vi "AutonCSV.vi"(0 "Auton Array":dbl[][](array[numeric]), 5 "MeasuredHeading":dbl, 7 "LeftEncoder":dbl, 9 "RightEncoder":dbl, 11 "Kinect Array":dbl[](array[numeric])) -> (2 "Z Wrist Right out":dbl, 3 "Z Wrist Left out":dbl, 4 "Left Drive":dbl, 6 "Right Drive":dbl)   [LabVIEW 2011]
uses:
  <vilib>/addons/Kinect/Skeleton Vertex Index.ctl
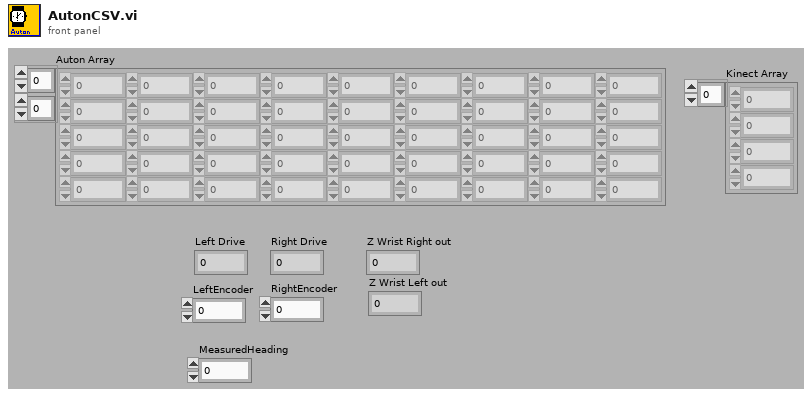
[diagram p1: front panel]
types:
  T1 = typedef "Skeleton Vertex Index.ctl" = i32
  T2 = cluster{"RightAxis":dbl, "LeftAxis":dbl, "RightHead":bool, "Left Head":bool, "Left Leg Out":bool, "Left Leg Forward":bool, "Left Leg Back":bool, "Right Leg Out":bool, "Right Leg Forward":bool, "Right Leg Back":bool}
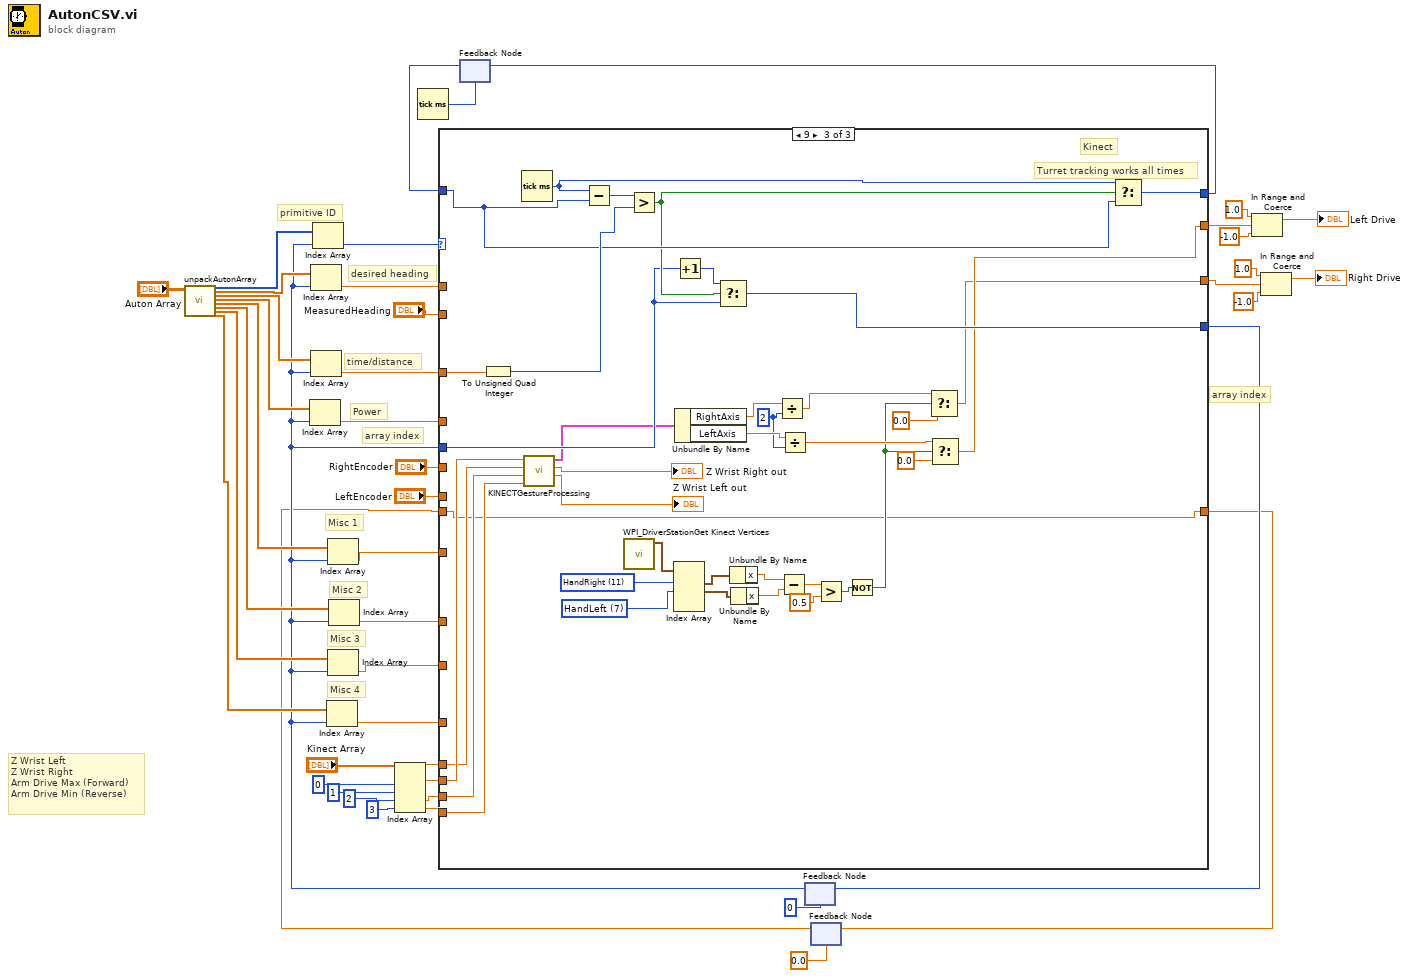
[diagram p0: block diagram]
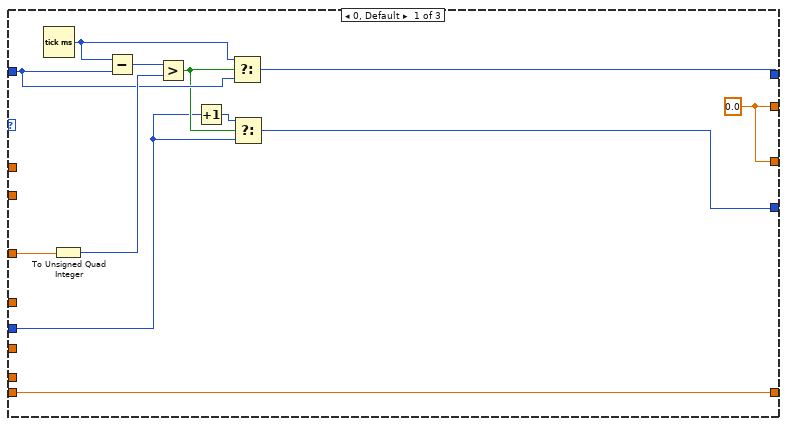
[diagram p2: hidden frame]
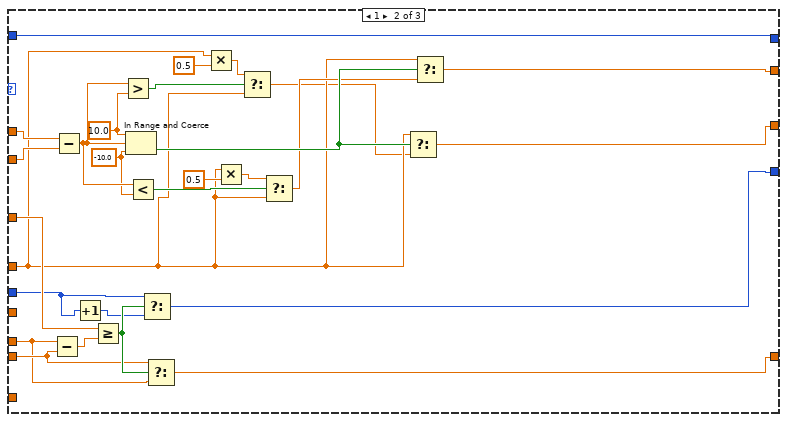
[diagram p3: hidden frame]
diagram:
  # "Misc 4"
  # "Misc 3"
  # "Misc 2"
  # "Misc 1"
  # "Z Wrist Left\nZ Wrist Right\nArm Drive Max (Forward)\nArm Drive Min (Reverse)"
  # "array index"
  # "array index"
  # "Power"
  # "desired heading"
  # "primitive ID"
  # "time/distance"
  n1 = call "unpackAutonArray.vi"("all rows"="Auton Array") -> ("Primitive"=w45:i16[], "Desired Heading"=w24:dbl[], "Time/Distance"=w23:dbl[], "Power"=w22:dbl[], "Misc 1"=w21:dbl[], "Misc 2"=w20:dbl[], "Misc 3"=w19:dbl[], "Misc 4"=w18:dbl[])  [unwired: 1 in, 18 out]
  n2 = Index Array(array="Kinect Array", index #1=0 ("index"), index #2=1 ("index"), index #3=2 ("index"), index #4=3 ("index")) -> (element #1=w7:dbl, element #2=w6:dbl, element #3=w5:dbl, element #4=w4:dbl)
  n3 = Tick Count (ms)() -> (millisecond timer value=w40:u32)
  n4 = feedback #1(w40) -> (w44:u32)
  n5 = feedback #2(0) -> (w16:i32)
  n6 = Index Array(array=w22, index=w16) -> (element=w42:dbl)
  n7 = Index Array(array=w24, index=w16) -> (element=w29:dbl)
  n8 = Index Array(array=w23, index=w16) -> (element=w43:dbl)
  n9 = Index Array(array=w45, index=w16) -> (element=w26:i16)
  n10 = Index Array(array=w18, index=w16) -> (element=w17:dbl)
  n11 = Index Array(array=w21, index=w16) -> (element=w25:dbl)
  n12 = Index Array(array=w19, index=w16) -> (element=w14:dbl)
  n13 = Index Array(array=w20, index=w16) -> (element=w15:dbl)
  n14 = feedback #3(0.0) -> (w2:dbl)
  n15 = case shown="9" w26 {
    tunnel: [w50 w81 w115] -> w27
    tunnel: w16 -> [w51 w61 w116]
    tunnel: [w58 w63 w123] -> w30
    tunnel: w44 -> [w55 w63 w120]
    tunnel: w43 -> [w48 w83 w114]
    tunnel: w29 -> [_ w80 _]
    tunnel: [w49 w77 w103] -> w38
    tunnel: [w49 w76 w102] -> w31
    tunnel: w42 -> [_ w65 _]
    tunnel: "LeftEncoder" -> [_ w59 _]
    tunnel: "MeasuredHeading" -> [_ w79 _]
    tunnel: w25 -> [_ _ _]
    tunnel: w17 -> [_ _ _]
    tunnel: w15 -> [_ _ _]
    tunnel: w14 -> [_ _ _]
    tunnel: "RightEncoder" -> [_ _ _]
    tunnel: w7 -> [_ _ w89]
    tunnel: w6 -> [_ _ w90]
    tunnel: w5 -> [_ _ w113]
    tunnel: w4 -> [_ _ w112]
    tunnel: w2 -> [w47 w60 w86]
    tunnel: [w47 w85 w86] -> w1
    frame 0, Default {
      w49 = 0.0 ("Numeric")
      n16 = Tick Count (ms)() -> (millisecond timer value=w54:u32)
      n17 = To Unsigned Quad Integer(1:w48) -> (0:w56:u64)
      n18 = Subtract(x=w54, y=w55) -> (x-y=w57:u32)
      n19 = Greater?(x=w57, y=w56) -> (0:w53:bool)
      n20 = Increment(x=w51) -> (x+1=w52:i32)
      n21 = Select(t=w54, s=w53, f=w55) -> (s? t:f=w58:u32)
      n22 = Select(t=w52, s=w53, f=w51) -> (s? t:f=w50:i32)
    }
    frame 1 {
      w73 = -10.0 ("lower limit")
      w75 = 10.0 ("upper limit")
      n23 = Subtract(x=w59, y=w60) -> (x-y=w84:dbl)
      n24 = Subtract(x=w80, y=w79) -> (x-y=w74:dbl)
      n25 = Increment(x=w61) -> (x+1=w62:i32)
      n26 = Greater Or Equal?(x=w83, y=w84) -> (x >= y?=w82:bool)
      n27 = Greater?(x=w74, y=w75) -> (0:w68:bool)
      n28 = In Range and Coerce(upper limit=w75, x=w74, lower limit=w73) -> (In Range?=w78:bool)  [unwired: 1 out]
      n29 = Less?(x=w74, y=w73) -> (x < y?=w72:bool)
      n30 = Select(t=w61, s=w82, f=w62) -> (s? t:f=w81:i32)
      n31 = Select(t=w60, s=w82, f=w59) -> (s? t:f=w85:dbl)
      n32 = Multiply(x=w65, y=0.5) -> (x*y=w67:dbl)
      n33 = Multiply(x=w65, y=0.5) -> (x*y=w70:dbl)
      n34 = Select(t=w67, s=w68, f=w65) -> (s? t:f=w64:dbl)
      n35 = Select(t=w70, s=w72, f=w65) -> (s? t:f=w69:dbl)
      n36 = Select(t=w65, s=w78, f=w64) -> (s? t:f=w76:dbl)
      n37 = Select(t=w65, s=w78, f=w69) -> (s? t:f=w77:dbl)
    }
    frame 9 {
      w91 = T1 7 items=["HipCenter", "Spine", "ShoulderCenter", "Head", "ShoulderLeft", "ElbowLeft", "WristLeft", "HandLeft", "ShoulderRight", "ElbowRight", "WristRight", "HandRight", "HipLeft", "KneeLeft", "AnkleLeft", "FootLeft", "HipRight", "KneeRight", "AnkleRight", "FootRight"] ("Skeleton Joints")
      w93 = T1 11 items=["HipCenter", "Spine", "ShoulderCenter", "Head", "ShoulderLeft", "ElbowLeft", "WristLeft", "HandLeft", "ShoulderRight", "ElbowRight", "WristRight", "HandRight", "HipLeft", "KneeLeft", "AnkleLeft", "FootLeft", "HipRight", "KneeRight", "AnkleRight", "FootRight"] ("Skeleton Joints")
      w108 = 2
      # "Kinect"
      # "Turret tracking works all times"
      n38 = To Unsigned Quad Integer(1:w114) -> (0:w121:u64)
      n39 = Tick Count (ms)() -> (millisecond timer value=w119:u32)
      n40 = call "KINECTGestureProcessing.vi"("Z Wrist Right in"=w90, "Z Wrist Left in"=w89, "Arm Drive in Max (Forward)"=w113, "Arm Drive in Min (Reverse)"=w112) -> ("Joystick Data"=w111:T2, "Z Wrist Right out"=→"Z Wrist Right out":dbl, "Z Wrist Left out"=→"Z Wrist Left out":dbl)  [unwired: 2 in]
      n41 = Subtract(x=w119, y=w120) -> (x-y=w122:u32)
      n42 = call <vilib>:"WPI_DriverStationGet Kinect Vertices.vi"() -> ("Skeleton Vertices"=w101:cluster{"x":sgl, "y":sgl, "z":sgl}[])  [unwired: 10 in, 1 out]
      n43 = Greater?(x=w122, y=w121) -> (0:w118:bool)
      n44 = Index Array(array=w101, index #1=w93, index #2=w91) -> (element #1=w94:cluster{"x":sgl, "y":sgl, "z":sgl}, element #2=w92:cluster{"x":sgl, "y":sgl, "z":sgl})  [unwired: 2 in, 2 out]
      n45 = Increment(x=w116) -> (x+1=w117:i32)
      n46 = Unbundle By Name(w111) -> ("RightAxis"=w110:dbl, "LeftAxis"=w109:dbl)
      n47 = Select(t=w117, s=w118, f=w116) -> (s? t:f=w115:i32)
      n48 = Unbundle By Name(w94) -> ("x"=w100:sgl)
      n49 = Unbundle By Name(w92) -> ("x"=w99:sgl)
      n50 = Divide(x=w110, y=w108) -> (x/y=w107:dbl)
      n51 = Subtract(x=w100, y=w99) -> (x-y=w98:sgl)
      n52 = Divide(x=w109, y=w108) -> (x/y=w106:dbl)
      n53 = Greater?(x=w98, y=sgl 0.5) -> (0:w96:bool)
      n54 = Not(x=w96) -> (.not. x?=w95:bool)
      n55 = Select(t=w107, s=w95, f=0.0) -> (s? t:f=w102:dbl)
      n56 = Select(t=w106, s=w95, f=0.0) -> (s? t:f=w103:dbl)
      n57 = Select(t=w119, s=w118, f=w120) -> (s? t:f=w123:u32)
    }
  }
  n58 = feedback-in #1(w30) -> ()
  n59 = feedback-in #2(w27) -> ()
  n60 = feedback-in #3(w1) -> ()
  n61 = In Range and Coerce(upper limit=1.0, x=w38, lower limit=-1.0) -> (coerced(x)=→"Left Drive":dbl)  [unwired: 1 out]
  n62 = In Range and Coerce(upper limit=1.0, x=w31, lower limit=-1.0) -> (coerced(x)=→"Right Drive":dbl)  [unwired: 1 out]
